vi "Calibration.vi"() -> ()   [LabVIEW 2021]
uses:
  <vilib>/Platform/TimedLoop/XDataNode/timing_clust.ctl
  <vilib>/Platform/TimedLoop/XDataNode/nitl_modes.ctl
  <vilib>/Platform/TimedLoop/XDataNode/wakeup.ctl
  <vilib>/platform/TimedLoop/XDataNode/XDataNode.xnode
  <vilib>/Platform/TimedLoop/XDataNode/XDNodeRunTimeDep.lvlib
panel:
  out "Gyroscope Bias (rad/s)":T1
  in  "Calibration Time (s)":dbl=5.0
  in  "Sampling Period (us)":i64=10000
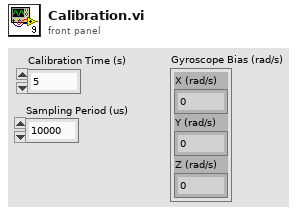
[diagram p1: front panel]
types:
  T1 = cluster{"X (rad/s)":dbl, "Y (rad/s)":dbl, "Z (rad/s)":dbl}
  T2 = typedef "Configuration.ctl" = cluster{"Accelerometer Bias":cluster{"X (m/s)":dbl, "Y (m/s)":dbl, "Z (m/s)":dbl}, "Gyroscope Bias":cluster{"X (m/s)":dbl, "Y (m/s)":dbl, "Z (m/s)":dbl}, "Steering Motor Gear Ratio":dbl, "Steering Pully Gear Ratio":dbl, "Steering Encoder CPR":dbl, "Steering Motor Max RPM":dbl, "Wheelbase (m)":dbl, "Fork Angle (rad)":dbl, "Balancing Controller":cluster{"Kp (/s)":dbl, "Kd (1)":dbl}, "Max Allowed Steering Angle (rad)":dbl, "Task Periods":cluster{"Emergency Stop (us)":i64, "IMU (us)":i64, "Steering Motor Encoder (us)":i64, "State Estimator (us)":i64, "Balancing Controller (us)":i64, "GNSS (us)":i64, "Logging (us)":i64, "Drive Motor (us)":i64}, "Drive Motor Gear Ratio":dbl}
  T3 = typedef "XDNodeRunTimeDep.lvlib/timing_clust.ctl" = cluster{"Expected End [f-1]":u64, "Actual End [f-1]":u64, "Finished Late? [f-1]":bool, "Expected End [i-1]":u64, "Actual End [i-1]":u64, "Finished Late? [i-1]":bool, "Expected Start [i]":u64, "Actual Start [i]":u64, "Expected Start [f]":u64, "Actual Start [f]":u64, "Source Name":string, "Structure Name":string, "Period":i64, "Deadline":i64, "Offset":i64, "Start":i64, "Priority":i32, "Timeout":i32, "Mode":T4, "Wakeup Reason":T5, "Error":errorcluster, "Source Type":string, "Secondary Source Type":string, "Global End Time":u64, "Global Start Time":u64, "Frame Duration":u64, "Iteration Duration":u64, "Assigned CPU":i32, "I/O Scan Engine Mode":u32}
  T4 = typedef "XDNodeRunTimeDep.lvlib/nitl_modes.ctl" = enum32{"No Change", "Process missed periods, maintain original phase", "Discard missed periods, maintain original phase", "Process missed periods, ignore original phase", "Discard missed periods, ignore original phase"}
  T5 = typedef "XDNodeRunTimeDep.lvlib/wakeup.ctl" = enum32{"Normal", "Aborted", "Asynchronous wakeup", "Timing source error", "Timed loop error", "Timeout"}
  T6 = typedef "IMU Handle.ctl" = cluster{"I2C address":u8}
  T7 = typedef "IMU Data.ctl" = cluster{"Gyroscope":cluster{"X (rad/s)":dbl, "Y (rad/s)":dbl, "Z (rad/s)":dbl}, "Accelerometer":cluster{"X (m/s^2)":dbl, "Y (m/s^2)":dbl, "Z (m/s^2)":dbl}, "Flag IMU":dbl}
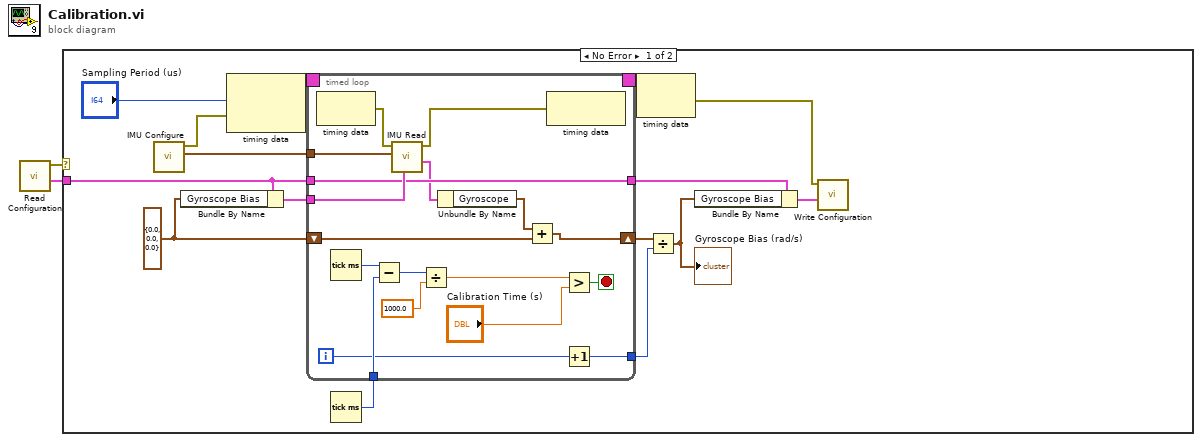
[diagram p0: block diagram]
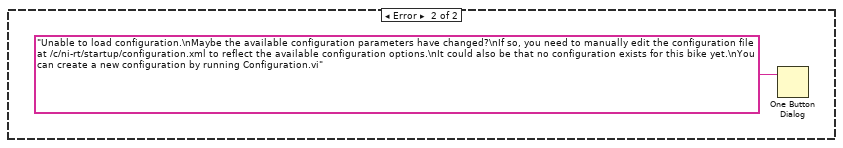
[diagram p2: hidden frame]
diagram:
  n1 = call "Read Configuration.vi"() -> ("Configuration"=w1:T2, "Error Out"=w2:errorcluster)  [unwired: 7 in, 3 out]
  n2 = case shown="No Error" w2 {
    tunnel: w1 -> [w9 _]
    frame No Error {
      w5 = T1 {"X (rad/s)"=0.0, "Y (rad/s)"=0.0, "Z (rad/s)"=0.0}
      n3 = call "IMU Configure.vi"() -> ("IMU Handle"=w12:T6, "Error Out"=w13:errorcluster)  [unwired: 10 in]
      n4 = Bundle By Name(cluster=w9, "Gyroscope Bias"=w5) -> (w10:T2)
      n5 = node-c288("Sampling Period (us)", w13) -> (w17:T3)
      n6 = Tick Count (ms)() -> (millisecond timer value=w14:u32)
      n7 = timed-loop {
        timing: w17 -> [_]
        timing-out: [_] -> w16
        tunnel: w14 -> [w34]
        tunnel: w12 -> [w28]
        shift-right: [w19] -> w4
        shift-left: w5 -> [w18]
        tunnel: [w24] -> w11
        tunnel: w10 -> [w23]
        tunnel: w9 -> [w22]
        tunnel: [w22] -> w8
        i -> [w25]
        stop <- w29 stop-if-true
        n8 = node-c288() -> (w27:errorcluster)  [unwired: 1 in]
        n9 = Tick Count (ms)() -> (millisecond timer value=w35:u32)
        n10 = Subtract(x=w35, y=w34) -> (x-y=w33:u32)
        n11 = call "IMU Read.vi"("Configuration"=w23, "IMU Handle"=w28, "Error In"=w27) -> ("IMU Data"=w21:T7, "Error Out"=w26:errorcluster)  [unwired: 6 in, 1 out]
        n12 = Divide(x=w33, y=1000.0) -> (x/y=w31:dbl)
        n13 = Unbundle By Name(w21) -> ("Gyroscope"=w20:T1)
        n14 = Add(x=w20, y=w18) -> (x+y=w19:T1)
        n15 = node-c288(w26) -> ()  [unwired: 1 out]
        n16 = Greater?(x=w31, y="Calibration Time (s)") -> (0:w29:bool)
        n17 = Increment(x=w25) -> (x+1=w24:i32)
      }
      n18 = node-c288(w16) -> (w6:errorcluster)
      n19 = Divide(x=w4, y=w11) -> (x/y=w3:T1)
      "Gyroscope Bias (rad/s)" <- w3
      n20 = Bundle By Name(cluster=w8, "Gyroscope Bias"=w3) -> (w7:T2)
      n21 = call "Write Configuration.vi"("Configuration"=w7, "Error In"=w6) -> ()  [unwired: 9 in, 1 out]
    }
    frame Error {
      n22 = One Button Dialog(message="Unable to load configuration.\nMaybe the available configuration parameters have changed?\nIf so, you need to manually edit the configuration file at /c/ni-rt/startup/configuration.xml to reflect the available configuration options.\nIt could also be that no configuration exists for this bike yet.\nYou can create a new configuration by running Configuration.vi") -> ()  [unwired: 1 in, 1 out]
    }
  }
